vi "RunInferenceAllOutput.vi"(4 "outputSizes":i32[](array[numeric]), 6 "inputIndex":i32, 7 "DLL path":path, 8 "error in (no error)":errorcluster, 9 "outputBuffer in":sgl[](array[numeric]), 10 "inputBuffer":sgl[](array[numeric]), 11 "session id in":i32) -> (0 "error out":errorcluster, 2 "outputBuffer":sgl[](array[numeric]), 3 "session id out":i32)   [LabVIEW 2017, in "ONNX Class Library.lvlib"]
doc: "/**\n * @brief Выполнить инференс (предсказание) модели\n * \n * Основная функция для получения предсказания от модели. Принимает входные данные,\n * передаёт их в нейросеть и записывает результат в выходной буфер.\n * \n * @param sessionId [IN] ID сессии\n * @param inputIndex [IN] Индекс входа (обычно 0 для моделей с одним входом)\n * @param inputBuffer [IN] Массив входных данных (тип должен соответствовать GetInputType)\n * @param inputSize [IN] Количество элементов во входном массиве\n * @param outputIndex [IN] Индекс выхода (обычно 0 для моделей с одним выходом)\n * @param outputBuffer [OUT] Массив для записи результатов (должен быть выделен в LabVIEW)\n * @param outputSize [IN] Размер выходного буфера в элементах\n * \n * @return int32: 0 при успешном выполнении инференса\n * @return int32: -1 при ошибке (сессия не загружена, неверные индексы, ошибка ONNX Runtime)\n * \n * @note Входные данные должны быть нормализованы так же, как при обучении модели\n * @note Размер входного массива должен соответствовать произведению всех размерностей shape\n * @note Выходной буфер должен быть достаточного размера (см. GetOutputShapeDim)\n * @note Функция блокирует выполнение до завершения инференса\n * \n * @example\n * // Для модели с входом [1, 10] и выходом [1, 3]:\n * float inputData[10] = {...};\n * float outputData[3];\n * RunInference(sessionId, 0, inputData, 10, 0, outputData, 3);\n */\nint RunInference(int sessionId, int inputIndex, float* inputBuffer, int inputSize, \n int outputIndex, float* outputBuffer, int outputSize);"
uses:
  ONNX Class Library.lvlib
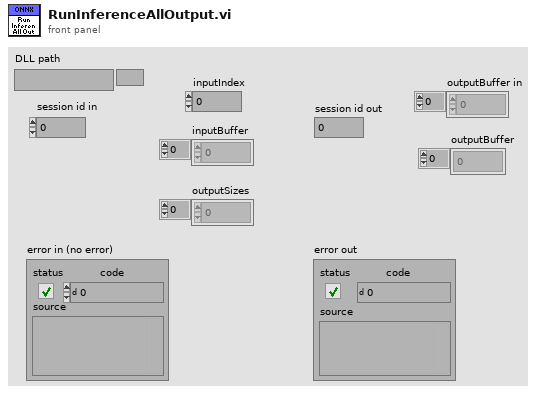
[diagram p1: front panel]
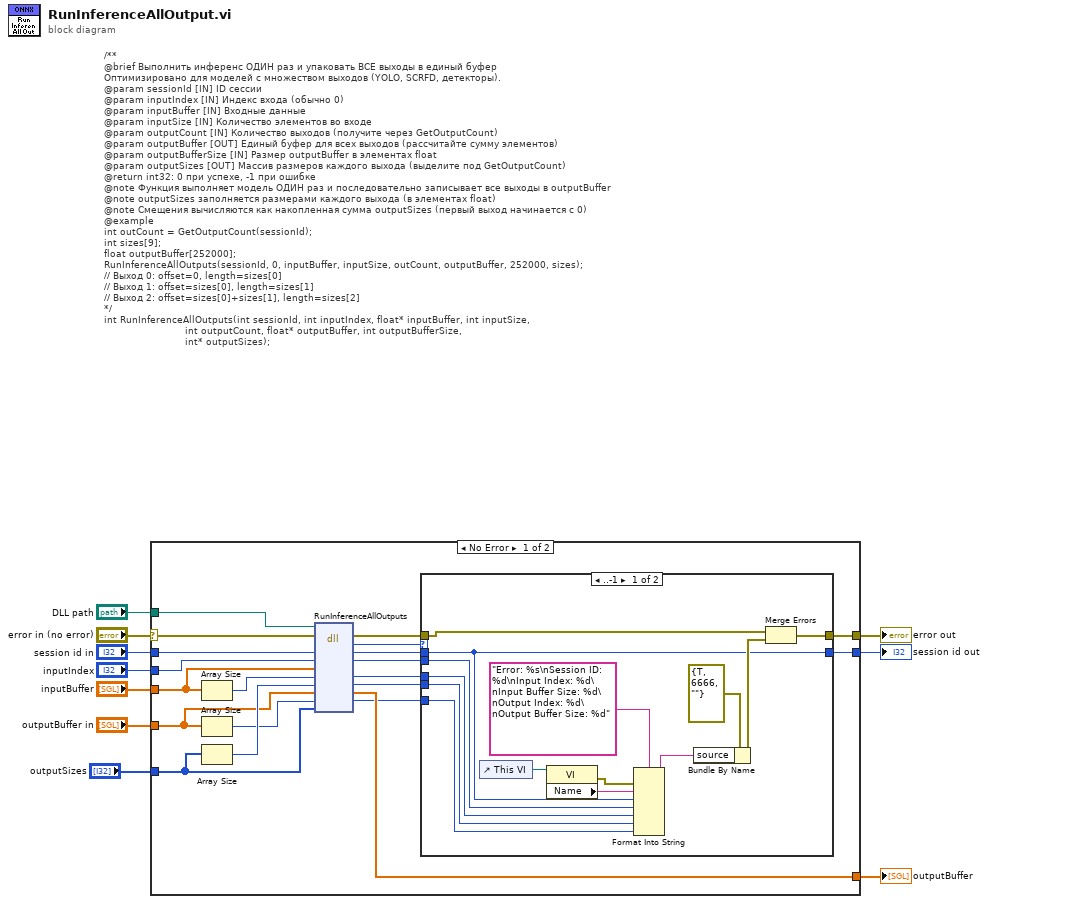
[diagram p0: block diagram]
diagram:
  # "/**\n@brief Выполнить инференс ОДИН раз и упаковать ВСЕ выходы в единый буфер\nОптимизировано для моделей с множеством выходов (YOLO, SCRFD, детекторы).\n@param sessionId [IN] ID сессии\n@param inputIndex [IN] Индекс входа (обычно 0)\n@param inputBuffer [IN] Входные данные\n@param inputSize [IN] Количество элементов во входе\n@param outputCount [IN] Количество выходов (получите через GetOutputCount)\n@param outputBuffer [OUT] Единый буфер для всех выходов (рассчитайте сумму элементов)\n@param outputBufferSize [IN] Размер outputBuffer в элементах float\n@param outputSizes [OUT] Массив размеров каждого выхода (выделите под GetOutputCount)\n@return int32: 0 при успехе, -1 при ошибке\n@note Функция выполняет модель ОДИН раз и последовательно записывает все выходы в outputBuffer\n@note outputSizes заполняется размерами каждого выхода (в элементах float)\n@note Смещения вычисляются как накопленная сумма outputSizes (первый выход начинается с 0)\n@example\nint outCount = GetOutputCount(sessionId);\nint sizes[9];\nfloat outputBuffer[252000];\nRunInferenceAllOutputs(sessionId, 0, inputBuffer, inputSize, outCount, outputBuffer, 252000, sizes);\n// Выход 0: offset=0, length=sizes[0]\n// Выход 1: offset=sizes[0], length=sizes[1]\n// Выход 2: offset=sizes[0]+sizes[1], length=sizes[2]\n*/\nint RunInferenceAllOutputs(int sessionId, int inputIndex, float* inputBuffer, int inputSize,\n                           int outputCount, float* outputBuffer, int outputBufferSize,\n                           int* outputSizes);"
  n1 = case shown="No Error" "error in (no error)" {
    selector: "error in (no error)" -> [w16 w48]
    tunnel: "session id in" -> [w30 w47]
    tunnel: "inputIndex" -> [w29 _]
    tunnel: "inputBuffer" -> [w28 _]
    tunnel: [w26 _] -> w7
    tunnel: [w22 w48] -> w6
    tunnel: [w21 w47] -> w5
    tunnel: "DLL path" -> [w15 _]
    tunnel: "outputSizes" -> [w13 _]
    tunnel: "outputBuffer in" -> [w12 _]
    frame No Error {
      n2 = Array Size(array=w28) -> (size(s)=w27:i32)
      n3 = Array Size(array=w12) -> (size(s)=w11:i32)
      n4 = Array Size(array=w13) -> (size(s)=w14:i32)
      n5 = dll-call lib="home/ivan/LabVIEWData/ONNX/LabVIEW-ONNX_Runtime/onnx_wrapper/unix64/libonnx_wrapper.so" fn="RunInferenceAllOutputs"(path in=w15, error in=w16, "sessionId"=w30, "inputIndex"=w29, "inputBuffer"=w28, "inputSize"=w27, "outputCount"=w14, "outputBuffer"=w12, "outputBufferSize"=w11, "outputSizes"=w13) -> (error out=w25:errorcluster, "return"=w24:i32, "sessionId"=w23:i32, "inputIndex"=w20:i32, "inputSize"=w19:i32, "outputCount"=w18:i32, "outputBuffer"=w26:sgl[], "outputBufferSize"=w17:i32)  [unwired: 3 in, 1 out]
      n6 = case shown="..-1" w24 {
        tunnel: w25 -> [w35 w46]
        tunnel: [w36 w46] -> w22
        tunnel: w23 -> [w37 w45]
        tunnel: [w37 w45] -> w21
        tunnel: w20 -> [w34 _]
        tunnel: w19 -> [w33 _]
        tunnel: w18 -> [w32 _]
        tunnel: w17 -> [w31 _]
        frame ..-1 {
          n7 = control-ref of="This VI"() -> (w41:refnum<vi>)
          n8 = property class="VI"(reference=w41) -> (error out=w38:errorcluster, "Name"=w40:string)  [unwired: 1 in, 1 out]
          n9 = Format Into String(format string="Error: %s\nSession ID: %d\nInput Index: %d\nInput Buffer Size: %d\nOutput Index: %d\nOutput Buffer Size: %d", error in=w38, w40, w37, w34, w33, w32, w31) -> (resulting string=w42:string)  [unwired: 1 in, 1 out]
          n10 = Bundle By Name(cluster=errorcluster {"status"=TRUE, "code"=6666, "source"=""} ("error out"), "source"=w42) -> (w43:errorcluster)
          n11 = Merge Errors(w35, w43) -> (w36:errorcluster)
        }
        frame 0.. {
        }
      }
    }
    frame Error {
    }
  }
  "error out" <- w6
  "session id out" <- w5
  "outputBuffer" <- w7
